vi "ParserCode.vi"(11 "ExampleParser in":refnum<class "ExampleParser.lvclass">) -> (2 "ParserCode":string, 3 "ExampleParser out":refnum<class "ExampleParser.lvclass">)   [LabVIEW 2022 SP3, in "ArgumentParser.lvlib" / "ExampleParser.lvclass"]
uses:
  ExampleParser.lvclass
  ExampleParser.lvclass/ExampleParser.ctl
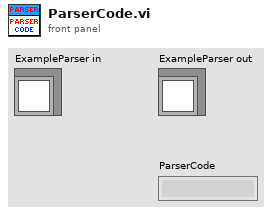
[diagram p1: front panel]
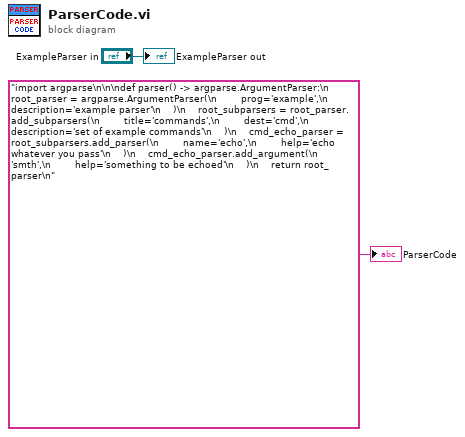
[diagram p0: block diagram]
diagram:
  "ExampleParser out" <- "ExampleParser in"
  "ParserCode" <- "import argparse\n\n\ndef parser() -> argparse.ArgumentParser:\n    root_parser = argparse.ArgumentParser(\n        prog='example',\n        description='example parser'\n    )\n    root_subparsers = root_parser.add_subparsers(\n        title='commands',\n        dest='cmd',\n        description='set of example commands'\n    )\n    cmd_echo_parser = root_subparsers.add_parser(\n        name='echo',\n        help='echo whatever you pass'\n    )\n    cmd_echo_parser.add_argument(\n        'smth',\n        help='something to be echoed'\n    )\n    return root_parser\n" ("ParserCode")
